vi "Read LV Version.vi"(8 "error in (no error)":errorcluster, 11 "VIP Install in":refnum<class "VIP Uninstall.lvclass">) -> (0 "error out":errorcluster, 2 "LV Version":string="14.0", 3 "VIP Install out":refnum<class "VIP Uninstall.lvclass">)   [LabVIEW 2014, in "VIP Uninstall.lvclass"]
uses:
  VIP Uninstall.lvclass
  VIP Uninstall.lvclass/VIP Uninstall.ctl
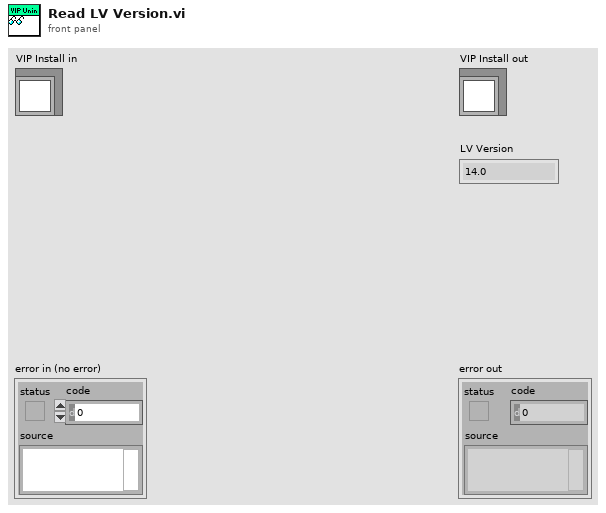
[diagram p1: front panel]
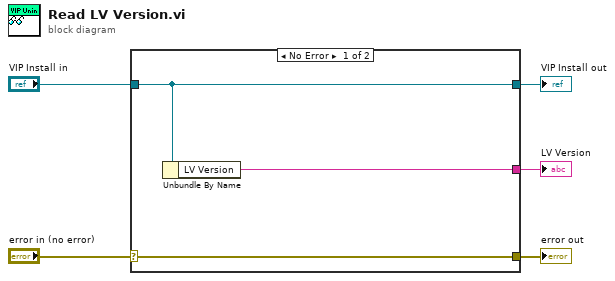
[diagram p0: block diagram]
diagram:
  n1 = case shown="No Error" "error in (no error)" {
    selector: "error in (no error)" -> [w8 w9]
    tunnel: [w8 w9] -> w4
    tunnel: [w7 w10] -> w2
    tunnel: "VIP Install in" -> [w7 w10]
    tunnel: [w6 _] -> w1
    frame No Error {
      n2 = Unbundle By Name(w7) -> ("LV Version"=w6:string)
    }
    frame Error {
    }
  }
  "error out" <- w4
  "VIP Install out" <- w2
  "LV Version" <- w1
